vi "Automotive ECU - Pedal Control.vi"() -> ()   [LabVIEW 2013]
doc: "Sample numeric display item."
uses:
  <vilib>/NI Veristand/Display Template Support/Display Template Support.llb/cluster_Screen Item Settings.ctl
  <vilib>/NI Veristand/Display Template Support/Display Template Support.llb/cluster_Graph Scale Settings.ctl
  <vilib>/NI Veristand/Display Template Support/Display Template Support.llb/cluster_Graph Plot Settings.ctl
  NationalInstruments.VeriStand.SystemStorage
  <vilib>/NI Veristand/Display Template Support/Display Template Support.llb/enum_Display Template Handler Minimal To Widget Msg.ctl
  <vilib>/NI Veristand/Display Template Support/Display Template Support.llb/enum_Display Template Handler Minimal To Workspace.ctl
  Support/Slide Parameters.ctl
  Support/PWM Object Parameters.ctl
  <vilib>/NI Veristand/Execution/Workspace/NI VeriStand - Get Single Channel Value.vi
  <vilib>/NI Veristand/Execution/Workspace/NI_VS Workspace ExecutionAPI.lvlib
panel:
  in  "Slide":dbl(slide) min=0.0 max=100.0 step=0.01 scale=0.0..100.0 scale format="%#5.2g"
  out "Label":string="Numeric"
  in  "NIVS.System Definition Root":refnum<k24>
  in  "NIVS.Gateway IP Address":string
  in  "Item.Data":T1
  # "yes, there is a transparent \ndecoration over the slider scale\nthis it to prevent the user from changing it manually."
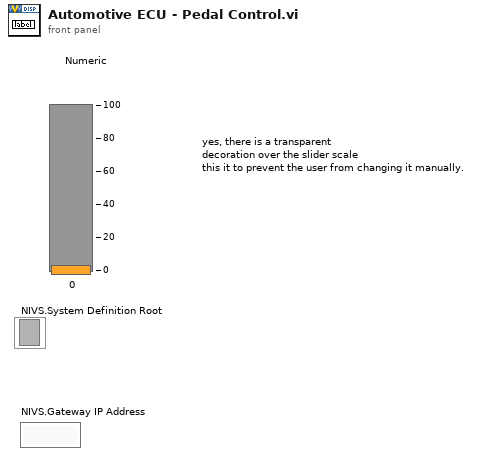
[diagram p1: front panel]
types:
  T1 = typedef "cluster_Screen Item Settings.ctl" = cluster{"Template VI":string, "Position X":i32, "Position Y":i32, "Custom":string, "Show Title Bar":bool, "ID":i32, "Always On Top":bool, "Allow Resize":bool, "Allow Minimize":bool, "Allow Close":bool, "Size to Screen":bool, "Screen.ID":i32, "State":enum16{"Normal", "New"}, "Title":string, "Window Bounds":cluster{"[0]":i16, "[1]":i16, "[2]":i16, "[3]":i16}, "Channel Ref":u64, "Unit":string, "Default Units?":bool, "Flash Limit?":bool, "Color 1":u32, "Color 2":u32, "Color 3":u32, "Color 4":u32, "Bck Color":u32, "Fore Color":u32, "Limit 1":dbl, "Limit 2":dbl, "Limit 3":dbl, "Limit 4":dbl, "Limit Mode 1":i32, "Limit Mode 2":i32, "Limit Mode 3":i32, "Limit Mode 4":i32, "Scale Precision":i32, "Scale Min":dbl, "Scale Max":dbl, "Format":i32, "Precision":i32, "Background Type":i32, "IDs":i32[], "Units":string[], "Labels":string[], "Scale Factor":dbl, "Scale Offset":dbl, "YScale Index":u32[], "XScale":T2, "YScales":T2[], "Plots":T3[], "Update Period":dbl, "History Length":dbl, "My.Ref":refnum<vi>, "Is Control?":bool, "Channel Paths":string[], "Custom Data":variant}
  T2 = typedef "cluster_Graph Scale Settings.ctl" = cluster{"Format":u8, "Precision":u8, "Fit":u8, "Label":string, "Use Default Label":bool, "Label Visible":bool, "Min":dbl, "Max":dbl}
  T3 = typedef "cluster_Graph Plot Settings.ctl" = cluster{"Bar Style":u8, "Fill To":i16, "Fill/PtColor":u32, "Line Style":u8, "Line Width":u8, "Color":u32, "Interp":u8, "Point Style":u8}
  T4 = typedef "enum_Display Template Handler Minimal To Workspace.ctl" = cluster{"Operation":enum16{"SetCustomData", "DeleteItem"}, "Data":variant}
  T5 = typedef "enum_Display Template Handler Minimal To Widget Msg.ctl" = enum16{"Stop", "LaunchConfigDialog"}
  T6 = typedef "Slide Parameters.ctl" = cluster{"Data cluster in":T7, "BG color":u32, "Initialized?":bool, "PWM Rails":dbl[], "Default Control Values":variant[]}
  T7 = typedef "PWM Object Parameters.ctl" = cluster{"RIO?":bool, "Label":string, "PWM Channel Path":cluster{"NodePathArray":string[], "Node Path":string}}
  T8 = typedef "NI_VS Workspace ExecutionAPI.lvlib/WorkspaceAPI.ctl" = refnum<k24>
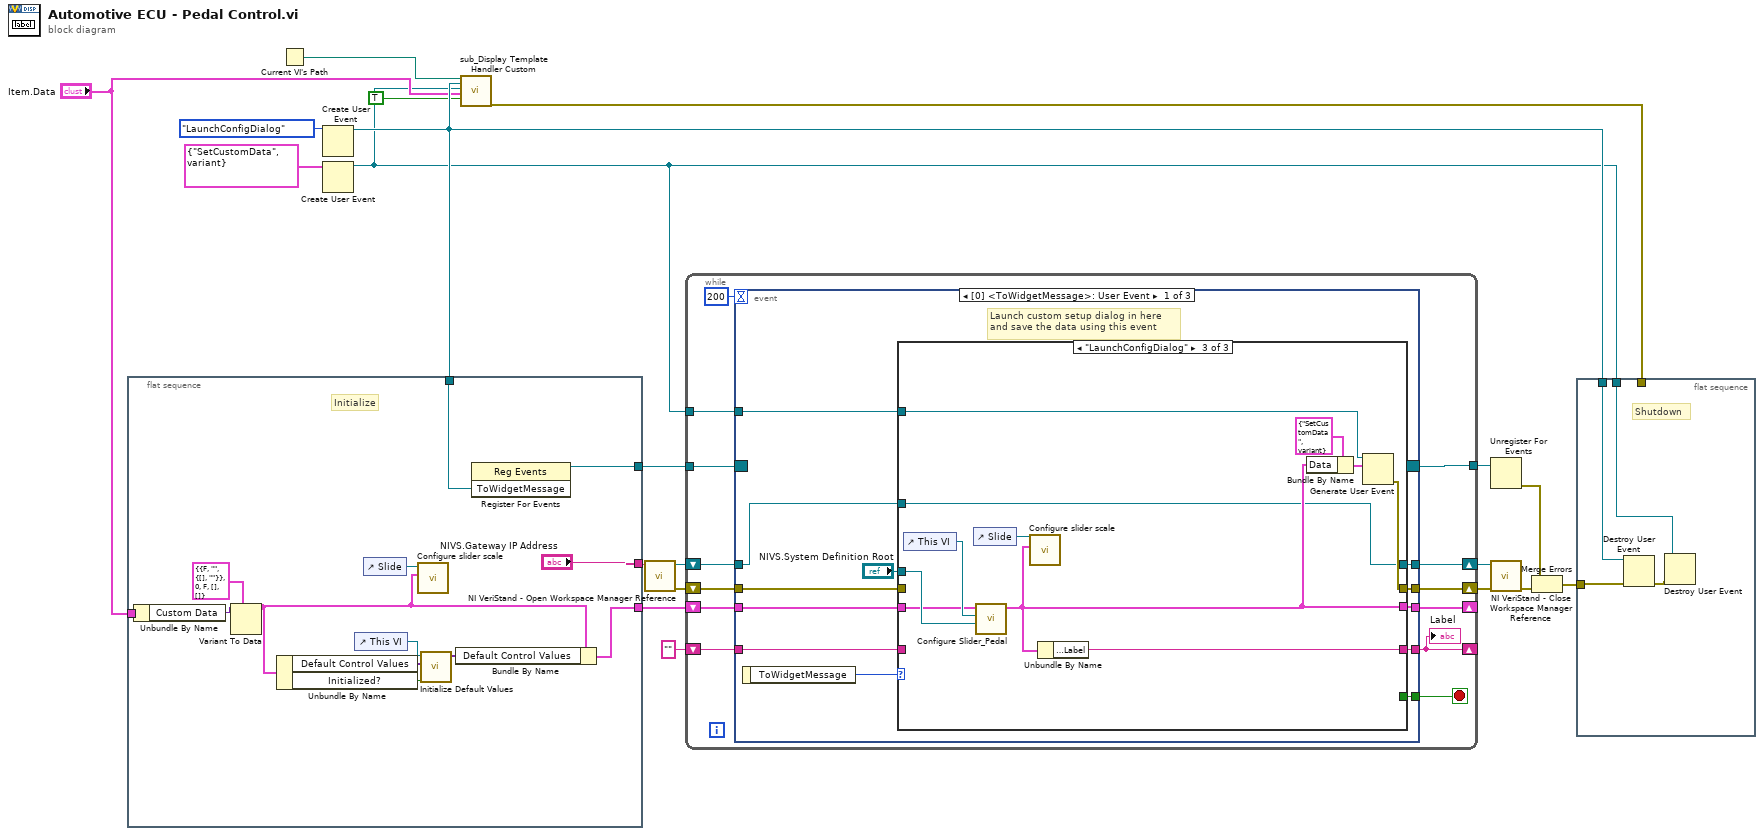
[diagram p0: block diagram]
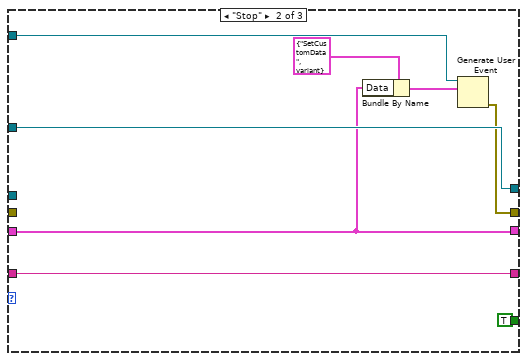
[diagram p3: hidden frame]
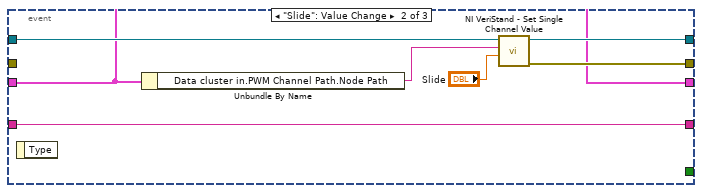
[diagram p4: hidden frame]
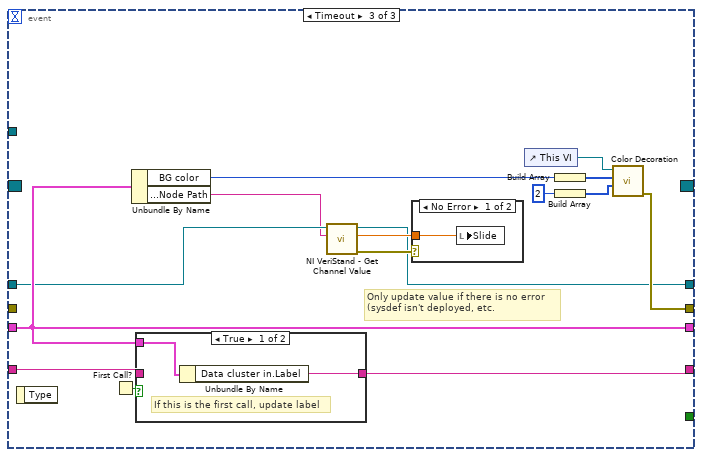
[diagram p5: hidden frame]
diagram:
  n1 = flat-sequence {
    tunnel: [w33] -> w18
    tunnel: w15 -> [w32]
    tunnel: "Item.Data" -> [w31]
    tunnel: [w22] -> w9
    tunnel: ["NIVS.Gateway IP Address"] -> w4
    frame #0 {
      # "Initialize"
      n2 = Unbundle By Name(w31) -> ("Custom Data"=w30:variant)
      n3 = Variant To Data(type=T6 {"Data cluster in"={"RIO?"=FALSE, "Label"="", "PWM Channel Path"={"NodePathArray"=[], "Node Path"=""}}, "BG color"=0, "Initialized?"=FALSE, "PWM Rails"=[], "Default Control Values"=[]} ("Slide Parameters"), Variant=w30) -> (data=w21:T6)  [unwired: 1 in, 1 out]
      n4 = Unbundle By Name(w21) -> ("Default Control Values"=w25:variant[], "Initialized?"=w23:bool)
      n5 = control-ref of="This VI"() -> (w24:refnum<vi>)
      n6 = control-ref of="Slide"() -> (w27:refnum<vi>)
      n7 = call "Configure slider scale.vi"("Slide Parameters"=w21, "Slide in"=w27) -> ()  [unwired: 8 in, 2 out]
      n8 = call "Initialize Default Values.vi"("Initialized?"=w23, "Default Control Values in"=w25, "VI in"=w24) -> ("Default Control Values out"=w26:variant[])  [unwired: 7 in, 1 out]
      n9 = Bundle By Name(cluster=w21, "Default Control Values"=w26) -> (w22:T6)
      n10 = register-events(w32) -> (reference out=w33:refnum<event-registration>)  [unwired: 2 in, 1 out]
    }
  }
  n11 = Current VI's Path() -> (path=w13:path)
  n12 = Create User Event(user event datatype=enum_Display_Template_Handler_Minimal_To_Widget_Msg."LaunchConfigDialog" ("ToWidgetMessage")) -> (user event=w15:refnum<user-event>)  [unwired: 1 in, 1 out]
  n13 = Create User Event(user event datatype=T4 {"Operation"=enum."SetCustomData", "Data"=variant} ("Data")) -> (user event=w11:refnum<user-event>)  [unwired: 1 in, 1 out]
  n14 = call <vilib>:"sub_Display Template Handler Custom.vi"("Parent.Path"=w13, "ToWidgetEvent"=w15, "ToWorkspace"=w11, "Item.Data"="Item.Data", "Resizable"=TRUE) -> ("error out"=w20:errorcluster)  [unwired: 14 in]
  n15 = call <vilib>:"NI VeriStand - Open Workspace Manager Reference.vi"("Gateway IP Address (\"\": localhost)"=w4) -> ("error out"=w7:errorcluster, "WorkspaceManager"=w8:T8)  [unwired: 9 in]
  n16 = while {
    tunnel: w18 -> [w46]
    tunnel: [w44] -> w17
    tunnel: w11 -> [w43]
    shift-right: [w35] -> _
    shift-left: w9 -> [w42]
    shift-right: [w39] -> w6
    shift-left: w8 -> [w41]
    shift-right: [w36] -> w5
    shift-left: w7 -> [w40]
    shift-right: [w37] -> _
    shift-left: "" ("Out") -> [w38]
    stop <- w45 stop-if-true
    n17 = event shown="[0] <ToWidgetMessage>: User Event" {
      selector: w46 -> [_ _ _]
      dyn-events: [_ _ _] -> w44
      timeout: 200 -> [_ _ _]
      tunnel: [w57 _ _] -> w45
      tunnel: w43 -> [w56 _ _]
      tunnel: w42 -> [w52 w84 w95]
      tunnel: w41 -> [w55 w85 w93]
      tunnel: w40 -> [w50 _ _]
      tunnel: [w54 w87 w89] -> w39
      tunnel: [w49 w88 w98] -> w36
      tunnel: [w48 w86 w102] -> w37
      tunnel: w38 -> [w47 w86 w101]
      tunnel: [w51 w84 w95] -> w35
      event User Event {
        # "Launch custom setup dialog in here\nand save the data using this event"
        n18 = event-data() -> ("ToWidgetMessage"=w58:T5)  [unwired: 1 out]
        n19 = case shown="\"LaunchConfigDialog\"" w58 {
          tunnel: [_ TRUE _] -> w57
          tunnel: w56 -> [_ w66 w79]
          tunnel: w55 -> [w62 w69 w71]
          tunnel: [w62 w69 w71] -> w54
          tunnel: "NIVS.System Definition Root" -> [_ _ w77]
          tunnel: w52 -> [w61 w65 w75]
          tunnel: [w61 w65 w72] -> w51
          tunnel: w50 -> [w59 _ _]
          tunnel: [w59 w64 w78] -> w49
          tunnel: [w60 w63 w74] -> w48
          tunnel: w47 -> [w60 w63 _]
          frame Default {
          }
          frame "Stop" {
            n20 = Bundle By Name(cluster=T4 {"Operation"=enum."SetCustomData", "Data"=variant} ("event data"), "Data"=w65) -> (w67:T4)
            n21 = Generate User Event(user event=w66, event data cluster=w67) -> (error out=w64:errorcluster)  [unwired: 2 in, 1 out]
          }
          frame "LaunchConfigDialog" {
            n22 = control-ref of="This VI"() -> (w76:refnum<vi>)
            n23 = control-ref of="Slide"() -> (w73:refnum<vi>)
            n24 = call "Configure Slider_Pedal.vi"("NIVS.System Definition Root"=w77, "VI Reference"=w76, "Slide Parameters In"=w75) -> ("Slide Parameters Out"=w72:T6)  [unwired: 7 in, 1 out]
            n25 = call "Configure slider scale.vi"("Slide Parameters"=w72, "Slide in"=w73) -> ()  [unwired: 8 in, 2 out]
            n26 = Unbundle By Name(w72) -> ("Data cluster in.Label"=w74:string)
            n27 = Bundle By Name(cluster=T4 {"Operation"=enum."SetCustomData", "Data"=variant} ("event data"), "Data"=w72) -> (w81:T4)
            n28 = Generate User Event(user event=w79, event data cluster=w81) -> (error out=w78:errorcluster)  [unwired: 2 in, 1 out]
          }
        }
      }
      event "Slide": Value Change {
        n29 = event-data() -> ()  [unwired: 2 out]
        n30 = Unbundle By Name(w84) -> ("Data cluster in.PWM Channel Path.Node Path"=w82:string)
        n31 = call <vilib>:"NI VeriStand - Set Single Channel Value.vi"("Value"="Slide", "Channel"=w82, "WorkspaceManager in"=w85) -> ("error out"=w88:errorcluster, "WorkspaceManager out"=w87:T8)  [unwired: 7 in]
      }
      event Timeout {
        # "Only update value if there is no error\n(sysdef isn't deployed, etc."
        n32 = event-data() -> ()  [unwired: 2 out]
        n33 = First Call?() -> (First Call?: T/F=w103:bool)
        n34 = Unbundle By Name(w95) -> ("BG color"=w94:u32, "Data cluster in.PWM Channel Path.Node Path"=w92:string)
        n35 = case shown="True" w103 {
          tunnel: w101 -> [_ w107]
          tunnel: [w105 w107] -> w102
          tunnel: w95 -> [w106 _]
          frame True {
            # "If this is the first call, update label"
            n36 = Unbundle By Name(w106) -> ("Data cluster in.Label"=w105:string)
          }
          frame False {
            # "If this is the first call, update label"
          }
        }
        n37 = call-poly <vilib>:"NI VeriStand - Get Channel Value.vi"("Channel"=w92, "WorkspaceManager in"=w93) -> ("error out"=w91:errorcluster, "Value"=w90:dbl, "WorkspaceManager out"=w89:T8)  [unwired: 7 in]
        n38 = case shown="No Error" w91 {
          tunnel: w90 -> [w104 _]
          frame No Error {
            n39 = local write "Slide"(w104) -> ()
          }
          frame Error {
          }
        }
        n40 = control-ref of="This VI"() -> (w100:refnum<vi>)
        n41 = Build Array(w94) -> (w99:u32[])
        n42 = Build Array(u32 2 ("BG color")) -> (w97:u32[])
        n43 = call "Color Decoration.vi"("VI reference"=w100, "Color Array"=w99, "Index Array"=w97) -> ("error out"=w98:errorcluster)  [unwired: 7 in]
      }
    }
    "Label" <- w37
  }
  n44 = Unregister For Events(event registration refnum=w17) -> (error out=w16:errorcluster)  [unwired: 1 in]
  n45 = call <vilib>:"NI VeriStand - Close Workspace Manager Reference.vi"("error in (no error)"=w5, "WorkspaceManager"=w6) -> ("error out"=w1:errorcluster)  [unwired: 9 in]
  n46 = Merge Errors(w16, w1) -> (w2:errorcluster)
  n47 = flat-sequence {
    tunnel: w20 -> [_]
    tunnel: w2 -> [w110]
    tunnel: w15 -> [w111]
    tunnel: w11 -> [w108]
    frame #0 {
      # "Shutdown"
      n48 = Destroy User Event(user event=w111, error in=w110) -> (error out=w109:errorcluster)
      n49 = Destroy User Event(user event=w108, error in=w109) -> ()  [unwired: 1 out]
    }
  }
